vi "Rx Channel Config Page.vi"(8 "error in (no error)":errorcluster, 11 "Node Ptr":T1 format="%.0x") -> (0 "error out":errorcluster)   [LabVIEW 2019, in "UDP-Custom-Device System Explorer.lvlib"]
uses:
  UDP-Custom-Device System Explorer.lvlib
  <vilib>/NI VeriStand/Custom Device API/Custom Device Item Ref.ctl
  Shared/Constants.vi
  <vilib>/NI VeriStand/Custom Device API/Set Item Property (Boolean).vi
  <vilib>/NI VeriStand/Custom Device API/Set Item Property (U32).vi
  <vilib>/NI VeriStand/Custom Device API/Custom Device API.lvlib
  Property Accessors/Shared Channel Accessors.lvlib
  <vilib>/NI VeriStand/Custom Device Tools/Custom Device Utility Library/Custom Device Utility Library.lvlib
  Shared/UDP-Custom-Device Shared.lvlib
panel:
  in  "Append To Channels":bool
  in  "Instances To Create":u32=1 min=1 step=1
  out "Imported Channel Configuration":i32[](listbox) caption="Channels"
  in  "Channel Configuration File":path
  in  "Description":string
  out "Name":string
  in  "SHDocVw.IWebBrowser":refnum<k7>(container)
  in  "General Header":cluster{"Section Name":string}={"Section Name"="Channel Configuration"}
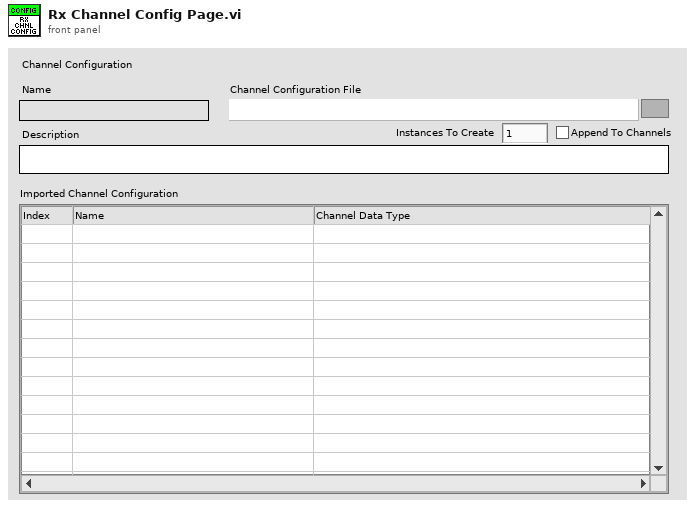
[diagram p1: front panel]
types:
  T1 = typedef "Custom Device API.lvlib/Custom Device Item Ref.ctl" = u64
  T2 = typedef "Custom Device API.lvlib/Custom Device Commands.ctl" = enum16{"Default", "Item renamed", "Shutdown", "Dynamic button pressed"}
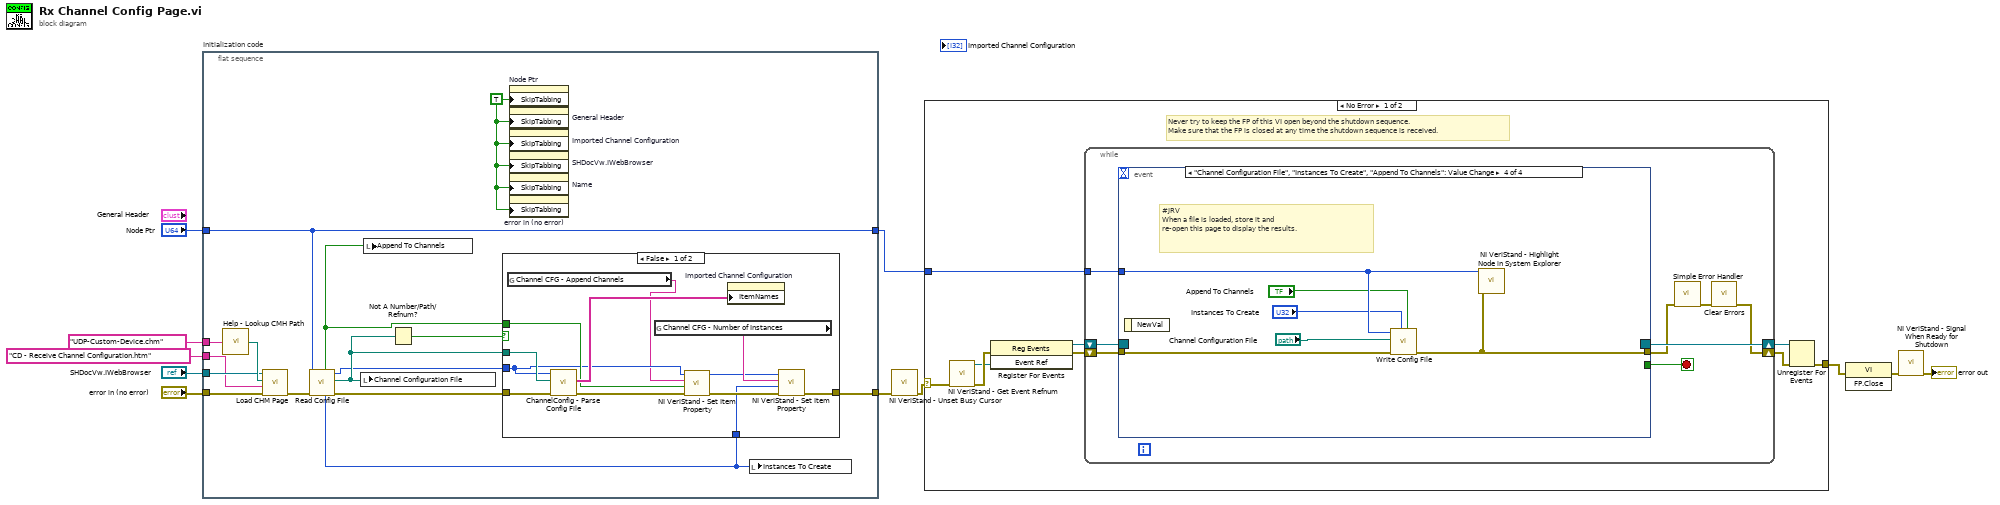
[diagram p0: block diagram]
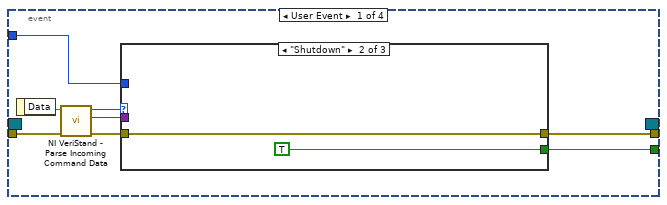
[diagram p3: hidden frame]
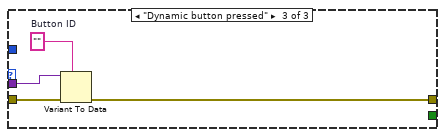
[diagram p5: hidden frame]
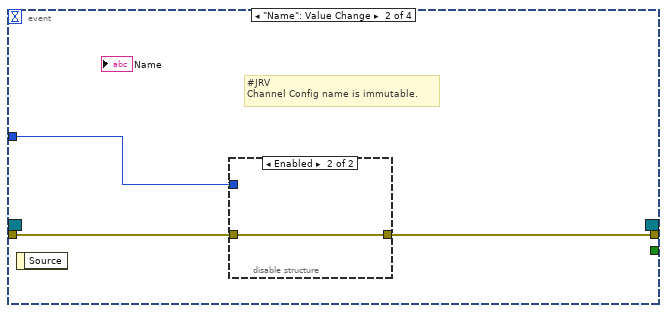
[diagram p6: hidden frame]
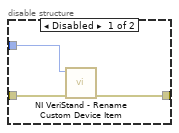
[diagram p7: hidden frame]
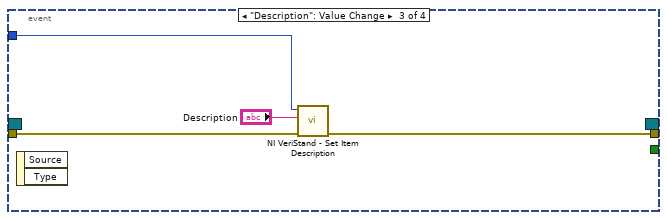
[diagram p8: hidden frame]
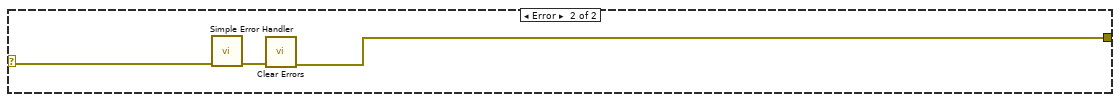
[diagram p9: hidden frame]
diagram:
  n1 = flat-sequence "Initialization code" {
    tunnel: "error in (no error)" -> [w25]
    tunnel: "Node Ptr" -> [w12]
    tunnel: [w20] -> w7
    tunnel: [w12] -> w4
    tunnel: "SHDocVw.IWebBrowser" -> [w24]
    tunnel: "CD - Receive Channel Configuration.htm" ("CD_CHM_Section") -> [w22]
    tunnel: "UDP-Custom-Device.chm" ("CD_CHM_FileName") -> [w23]
    frame #0 {
      w16 = TRUE ("Skip When Tabbing")
      n2 = call "Help - Lookup CMH Path.vi"("Main CMH File"=w23) -> ("Compiled CMH Path"=w26:path)
      n3 = call <vilib>:"Load CHM Page.vi"("error in (no error)"=w25, "HTML File"=w22, "Compiled CHM Path"=w26, "Web Browser Reference"=w24) -> ("error out"=w21:errorcluster)  [unwired: 7 in]
      n4 = call "Read Config File.vi"("error in (no error)"=w21, "Node Ptr"=w12) -> ("error out"=w19:errorcluster, "Config File"=w17:path, "Node Ptr out"=w13:T1, "NumberOfInstances"=w15:u32, "AppendToChannels"=w14:bool)  [unwired: 5 in]
      n5 = local write "Channel Configuration File"(w17) -> ()
      n6 = local write "Append To Channels"(w14) -> ()
      n7 = Not A Number/Path/Refnum?(number/path/refnum=w17) -> (NaN/Path/Refnum?=w18:bool)
      n8 = case shown="False" w18 {
        tunnel: [w35 w38] -> w20
        tunnel: w19 -> [w36 w38]
        tunnel: w17 -> [w37 _]
        tunnel: w13 -> [w28 _]
        tunnel: w15 -> [w30 _]
        tunnel: w14 -> [w29 _]
        frame False {
          n9 = global read "Constants.vi" "Channel CFG - Append Channels"() -> (w27:string)
          n10 = call "ChannelConfig - Parse Config File.vi"("error in (no error)"=w36, "Config Path"=w37, "Node Ptr"=w28) -> ("error out"=w35:errorcluster, "Channel Configuration"=w34:string[][])  [unwired: 6 in, 1 out]
          n11 = global read "Constants.vi" "Channel CFG - Number of Instances"() -> (w32:string)
          n12 = call-poly <vilib>:"NI VeriStand - Set Item Property.vi"("Value"=w29, "Property Name"=w27, "Item Ref in"=w28) -> ("error out"=w33:errorcluster, "Item Ref out"=w31:T1)  [unwired: 6 in, 1 out]
          n13 = property on="Imported Channel Configuration" class="MCListbox (strict)"("ItemNames"=w34) -> ()  [unwired: 2 in, 2 out]
          n14 = call-poly <vilib>:"NI VeriStand - Set Item Property.vi"("error in (no error)"=w33, "Value"=w30, "Property Name"=w32, "Item Ref in"=w31) -> ()  [unwired: 5 in, 3 out]
        }
        frame True {
        }
      }
      n15 = property on="Node Ptr" class="DigNum (strict)"("SkipTabbing"=w16) -> ()  [unwired: 2 in, 2 out]
      n16 = property on="General Header" class="Clust (strict)"("SkipTabbing"=w16) -> ()  [unwired: 2 in, 2 out]
      n17 = property on="Imported Channel Configuration" class="MCListbox (strict)"("SkipTabbing"=w16) -> ()  [unwired: 2 in, 2 out]
      n18 = property on="SHDocVw.IWebBrowser" class="AXCont"("SkipTabbing"=w16) -> ()  [unwired: 2 in, 2 out]
      n19 = property on="Name" class="Str"("SkipTabbing"=w16) -> ()  [unwired: 2 in, 2 out]
      n20 = property on="error in (no error)" class="Clust (strict)"("SkipTabbing"=w16) -> ()  [unwired: 2 in, 2 out]
      n21 = local write "Instances To Create"(w15) -> ()
    }
  }
  n22 = call <vilib>:"NI VeriStand - Unset Busy Cursor.vi"("error in (no error)"=w7) -> ("error out"=w6:errorcluster)  [unwired: 10 out]
  n23 = case shown="No Error" w6 {
    selector: w6 -> [w39 w90]
    tunnel: [w44 w88] -> w11
    tunnel: w4 -> [w40 _]
    frame No Error {
      # "Never try to keep the FP of this VI open beyond the shutdown sequence.\nMake sure that the FP is closed at any time the shutdown sequence is received."
      n24 = call <vilib>:"NI VeriStand - Get Event Refnum.vi"("error in (no error)"=w39) -> ("error out"=w47:errorcluster, "Event Ref"=w43:refnum<user-event>)  [unwired: 9 out]
      n25 = register-events(error in=w47, w43) -> (reference out=w41:refnum<event-registration>, error out=w42:errorcluster)  [unwired: 1 in]
      n26 = while {
        tunnel: w40 -> [w51]
        shift-right: [w48] -> w45
        shift-left: w42 -> [w54]
        shift-right: [w55] -> w46
        shift-left: w41 -> [w53]
        stop <- w52 stop-if-true
        n27 = event shown="[3] \"Channel Configuration File\", \"Instances To Create\", \"Append To Channels\": Value Change" {
          selector: w53 -> [_ _ _ _]
          dyn-events: [_ _ _ _] -> w55
          timeout: _ -> [_ _ _ _]
          tunnel: w54 -> [w63 w73 w81 w86]
          tunnel: [w59 _ _ _] -> w52
          tunnel: [w58 w71 w78 w85] -> w50
          tunnel: w51 -> [w57 w72 w80 w87]
          event User Event {
            n28 = event-data() -> ("Data"=w62:string)  [unwired: 1 out]
            n29 = call <vilib>:"NI VeriStand - Parse Incoming Command Data.vi"("error in (no error)"=w63, "Incoming data"=w62) -> ("error out"=w61:errorcluster, "Outgoing data"=w56:variant, "Action"=w60:T2)  [unwired: 7 out]
            n30 = case shown="\"Shutdown\"" w60 {
              tunnel: w61 -> [w64 w65 w70]
              tunnel: [_ TRUE _] -> w59
              tunnel: [w64 w65 w67] -> w58
              tunnel: w57 -> [_ _ _]
              tunnel: w56 -> [_ _ w69]
              frame "Default", Default {
              }
              frame "Shutdown" {
              }
              frame "Dynamic button pressed" {
                w68 = ""  # Button ID
                n31 = Variant To Data(error in=w70, type=w68, Variant=w69) -> (error out=w67:errorcluster)  [unwired: 1 out]
              }
            }
          }
          event "Name": Value Change {
            # "#JRV\nChannel Config name is immutable."
            n32 = event-data() -> ()  [unwired: 2 out]
            n33 = disable-structure shown="Enabled" {
              disable-tunnel: w73 -> [w76 w77]
              disable-tunnel: w72 -> [w75 _]
              disable-tunnel: [w74 w77] -> w71
              frame Disabled {
                n34 = call <vilib>:"NI VeriStand - Rename Custom Device Item.vi"("error in (no error)"=w76, "Item Ref in"=w75) -> ("error out"=w74:errorcluster)  [unwired: 7 in, 2 out]
              }
              frame Enabled {
              }
            }
          }
          event "Description": Value Change {
            n35 = event-data() -> ()  [unwired: 3 out]
            n36 = call <vilib>:"NI VeriStand - Set Item Description.vi"("error in (no error)"=w81, "Description"="Description", "Item Ref in"=w80) -> ("error out"=w78:errorcluster)  [unwired: 6 in, 2 out]
          }
          event "Channel Configuration File", "Instances To Create", "Append To Channels": Value Change {
            # "#JRV\nWhen a file is loaded, store it and\nre-open this page to display the results."
            n37 = event-data() -> ()  [unwired: 2 out]
            n38 = call "Write Config File.vi"("Append To Channels"="Append To Channels", "Instances To Create"="Instances To Create", "error in (no error)"=w86, "Config File"="Channel Configuration File", "Node Ptr"=w87) -> ("error out"=w85:errorcluster)  [unwired: 5 in, 1 out]
            n39 = call <vilib>:"NI VeriStand - Highlight Node in System Explorer.vi"("error in (no error)"=w85, "Item Ref in"=w87) -> ()  [unwired: 8 in, 2 out]
          }
        }
        n40 = call <vilib>:"Simple Error Handler.vi"("error in (no error)"=w50) -> ("error out"=w49:errorcluster)  [unwired: 1 in, 7 out]
        n41 = call <vilib>:"Clear Errors.vi"("error in (no error)"=w49) -> ("error out"=w48:errorcluster)  [unwired: 1 in, 5 out]
      }
      n42 = Unregister For Events(event registration refnum=w46, error in=w45) -> (error out=w44:errorcluster)
    }
    frame Error {
      n43 = call <vilib>:"Simple Error Handler.vi"("error in (no error)"=w90) -> ("error out"=w89:errorcluster)  [unwired: 1 in, 7 out]
      n44 = call <vilib>:"Clear Errors.vi"("error in (no error)"=w89) -> ("error out"=w88:errorcluster)  [unwired: 1 in, 5 out]
    }
  }
  n45 = invoke class="VI" method="FP.Close"(error in=w11) -> (error out=w10:errorcluster)  [unwired: 2 in, 2 out]
  n46 = call <vilib>:"NI VeriStand - Signal When Ready for Shutdown.vi"("error in (no error)"=w10) -> ("error out"=→"error out":errorcluster)  [unwired: 10 out]
